vi "Include_when_Saving.vi"(8 "error in (no error)":errorcluster, 11 "AB_Source_VI in":refnum<class "AB_Source_VI.lvclass">) -> (0 "error out":errorcluster, 2 "include":bool, 3 "AB_Source_VI out":refnum<class "AB_Source_VI.lvclass">)   [LabVIEW 2020, in "AB_Source_VI.lvclass"]
uses:
  <vilib>/AppBuilder/AB_Classes/Source/VI/AB_Source_VI.lvclass
  <vilib>/AppBuilder/AB_Classes/Source/VI/AB_Source_VI.lvclass/AB_Source_VI.ctl
  <vilib>/AppBuilder/AB_Classes/Source/AB_Source.lvclass
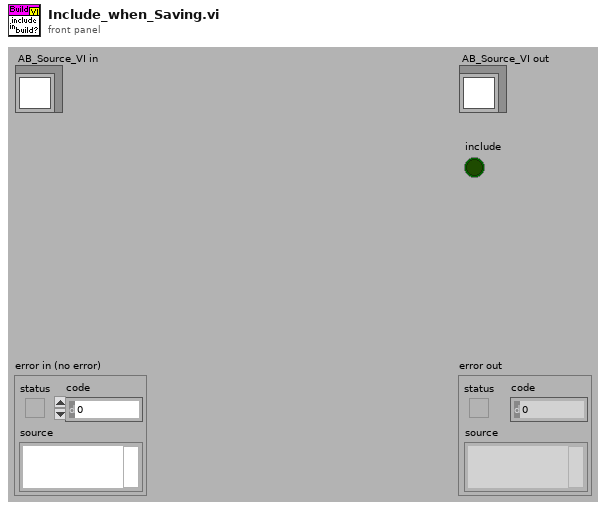
[diagram p1: front panel]
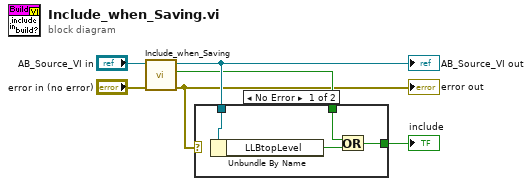
[diagram p0: block diagram]
diagram:
  n1 = call-parent "Include_when_Saving.vi"("error in (no error)"="error in (no error)", "AB_Source in"="AB_Source_VI in") -> ("error out"=w2:errorcluster, "include"=w3:bool, "AB_Source out"=w4:refnum<class "AB_Source_VI.lvclass">)  [unwired: 7 in]
  "error out" <- w2
  "AB_Source_VI out" <- w4
  n2 = case shown="No Error" w2 {
    tunnel: w4 -> [w10 _]
    tunnel: w3 -> [w8 _]
    tunnel: [w7 _] -> w1
    frame No Error {
      n3 = Unbundle By Name(w10) -> ("LLBtopLevel"=w9:bool)
      n4 = Or(x=w8, y=w9) -> (x .or. y?=w7:bool)
    }
    frame Error {
    }
  }
  "include" <- w1
